vi "OBDservice02.vi"(8 "错误输入（无错误）":errorcluster, 11 "diag ref out输入":T2 {"Diagostic Globals"."Fill Byte" format="%x"; "TesterPresent Message" format="%.0x"; "Selected I/O Mode" items=["CAN", "CAN FD", "CAN FD+BRS", "ECU Determined"]; "DoIP Protocol Version" items=["2010"=1, "2012"=2]; "RX_DL" items=["8"=8, "12"=12, "16"=16, "20"=20, "24"=24, "32"=32, "48"=48, "64"=64]; "TX_DL" items=["8"=8, "12"=12, "16"=16, "20"=20, "24"=24, "32"=32, "48"=48, "64"=64]; "I/O Mode" items=["CAN", "CAN FD", "CAN FD+BRS", "Not yet determined"]}) -> (0 "错误输出":errorcluster, 1 "success?":bool, 2 "冻结帧":T1(array[cluster]), 3 "diag ref out输出":T2 {"Diagostic Globals"."Fill Byte" format="%x"; "TesterPresent Message" format="%.0x"; "Selected I/O Mode" items=["CAN", "CAN FD", "CAN FD+BRS", "ECU Determined"]; "DoIP Protocol Version" items=["2010"=1, "2012"=2]; "RX_DL" items=["8"=8, "12"=12, "16"=16, "20"=20, "24"=24, "32"=32, "48"=48, "64"=64]; "TX_DL" items=["8"=8, "12"=12, "16"=16, "20"=20, "24"=24, "32"=32, "48"=48, "64"=64]; "I/O Mode" items=["CAN", "CAN FD", "CAN FD+BRS", "Not yet determined"]}, 5 "PIDs out":u8[](array[numeric]))   [LabVIEW 2018]
uses:
  <vilib>/Automotive Diagnostic Command Set/Diagnostic Transport.llb/Diag Reference.ctl
  <vilib>/Automotive Diagnostic Command Set/Diagnostic Transport.llb/Transport Protocol Selector.ctl
  <vilib>/Automotive Diagnostic Command Set/Diagnostic Transport.llb/DoIP Protocol Version.ctl
  <vilib>/Automotive Diagnostic Command Set/Diagnostic Transport.llb/Diag Globals.ctl
  <vilib>/Automotive Diagnostic Command Set/Diagnostic Protocols.llb/Diagnostic Trouble Code.ctl
  <vilib>/addons/Automotive Diagnostic Command Set/NI_Automotive Diagnostic Command Set.lvlib
panel:
  out "数组":bool[][](array[boolean])
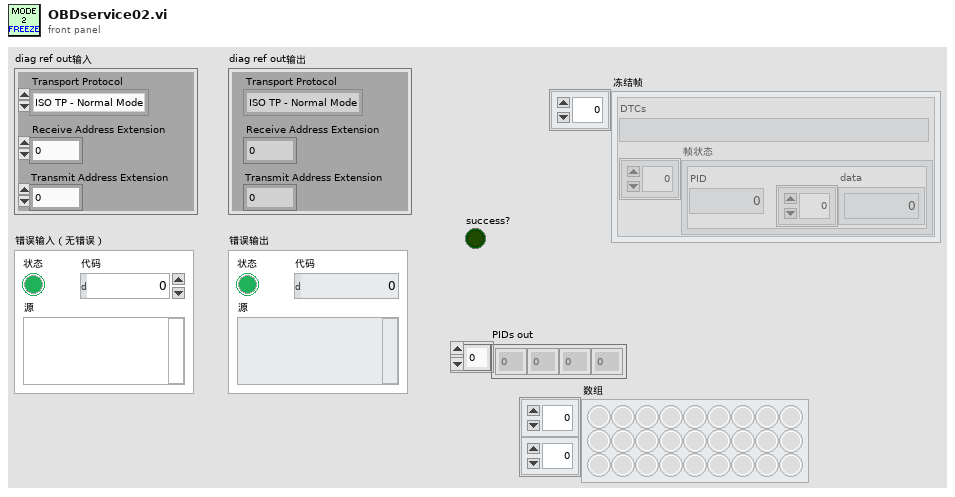
[diagram p1: front panel]
types:
  T1 = cluster{"DTCs":string, "帧状态":cluster{"PID":u8, "data":u8[]}[]}[]
  T2 = typedef "NI_Automotive Diagnostic Command Set.lvlib/Diag Reference.ctl" = cluster{"Diag CAN Handle":u32, "Transport Protocol":T3, "Receive Address Extension":u8, "Transmit Address Extension":u8, "Receive CAN Id":u32, "Transmit CAN Id":u32, "Log Frames ?":bool, "My TP Address":u8, "Other TP Address":u8, "T1":u16, "T2":u16, "T3":u16, "T4":u16, "Tx SN":u8, "Block Size":u8, "Rx SN":u8, "VW TP Initialized?":bool, "Tx block no":u8, "baud rate":u64, "Interface":string, "Channel Diag CAN Handle":u32, "UDP Connection ID":refnum<k16>, "TCP Connection ID":refnum<k5>, "Target IP Addr":u32, "Source Address":u16, "Target Address":u16, "Send Header NACK?":bool, "DLL Handle":u32, "NAD":u8, "Time Stamp read first":dbl, "Time Stamp read last":dbl, "Time Stamp write first":dbl, "Time Stamp write last":dbl, "Time Stamp write":dbl, "Time Stamp read":dbl, " I/O Mode":u32, "FD Baudrate":u64, "TX_DL":u16, "RX_DL":u16, "DoIP Protocol Version":T4, " Selected I/O Mode":u32, "TesterPresent Counter":u32, "TesterPresent Limit":u32, "TesterPresent Tick[ms]":i32, "TesterPresent RequireResponse?":bool, "TesterPresent Stored Ref?":bool, "TesterPresent Message":u8[], "TesterPresent Task Handle":i32, "TesterPresent Semaphore":T5, "Response Plausibility Check":u32, "Default Version?":bool, "Diagostic Globals":T6, "Session-based Properties?":bool}
  T3 = typedef "NI_Automotive Diagnostic Command Set.lvlib/Transport Protocol Selector.ctl" = enum16{"ISO TP - Normal Mode", "ISO TP - Mixed Mode", "VW TP 2.0", "Diagnostics on IP", "ISO TP LIN"}
  T4 = typedef "NI_Automotive Diagnostic Command Set.lvlib/DoIP Protocol Version.ctl" = u8
  T5 = typedef "Semaphore RefNum" = refnum<k1>
  T6 = typedef "NI_Automotive Diagnostic Command Set.lvlib/Diag Globals.ctl" = cluster{"Timeout FC (Bs)":u32, "Timeout CF (Cr)":u32, "Timeout Diag Command":u32, "Receive Block Size (BS)":u8, "Wait Time CF (STmin)":u8, "Max Waits (N_WFTmax)":u8, "Waits to Send (N_WAIT)":i32, "Time between Waits (TW)":u32, "Fill CAN Frames?":bool, "Fill Byte":u32, "Invalid Response as Error?":bool, "Max RspPending Count":u32, "VWTP Command Timeout":u32, "Transport Protocol":T3, "Diag CAN Handle":u32, "DLL Handle":u32, "Timeout RspPending":u32}
  T7 = cluster{"DTCs":string, "数组":cluster{"PID":u8, "data":u8[]}[]}
  T8 = typedef "Diagnostic Trouble Code.ctl" = cluster{"DTC":u32, "Status":u32, "Add Data":u32}
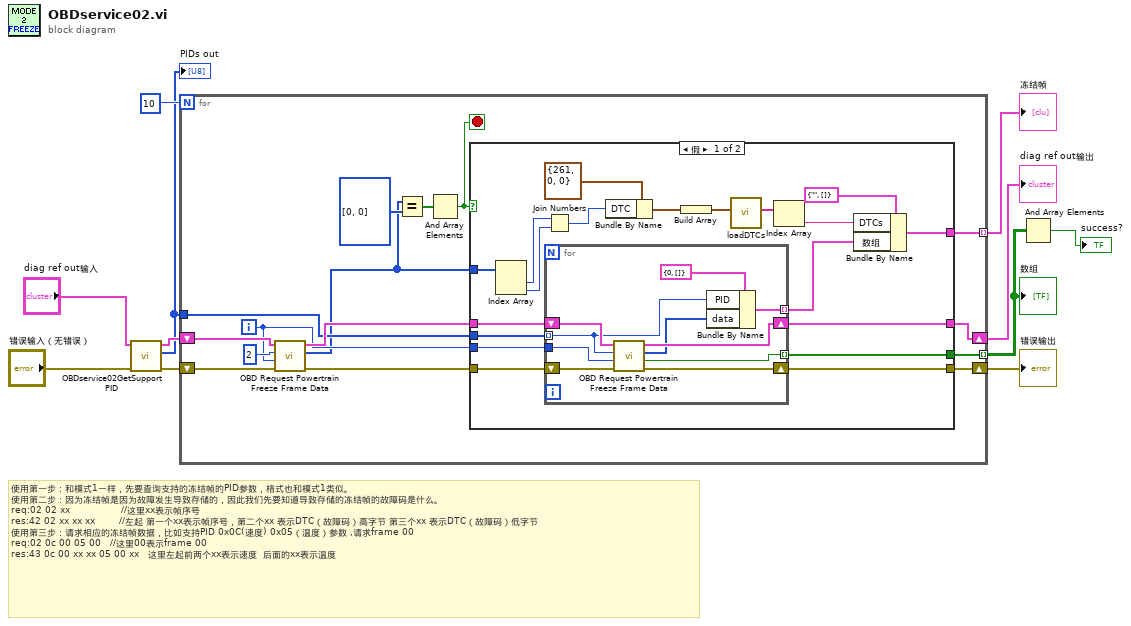
[diagram p0: block diagram]
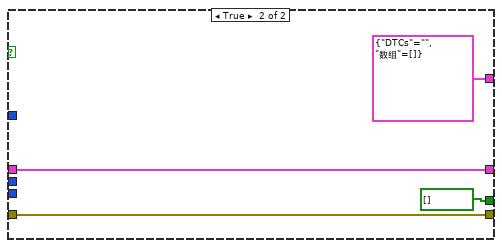
[diagram p2: hidden frame]
diagram:
  # "使用第一步：和模式1一样，先要查询支持的冻结帧的PID参数，格式也和模式1类似。\n使用第二步：因为冻结帧是因为故障发生导致存储的，因此我们先要知道导致存储的冻结帧的故障码是什么。\nreq:02 02 xx                 //这里xx表示帧序号\nres:42 02 xx xx xx        //左起 第一个xx表示帧序号，第二个xx 表示DTC（故障码）高字节 第三个xx 表示DTC（故障码）低字节\n使用第三步：请求相应的冻结帧数据，比如支持PID 0x0C(速度) 0x05（温度）参数 ,请求frame 00\nreq:02 0c 00 05 00   //这里00表示frame 00 \nres:43 0c 00 xx xx 05 00 xx   这里左起前两个xx表示速度  后面的xx表示温度"
  n1 = call "OBDservice02GetSupportPID.vi"("error in (no error) 2"="错误输入（无错误）", "diag ref in"="diag ref out输入") -> ("error out 2"=w8:errorcluster, "PIDs out"=w6:u8[], "diag ref out 2"=w9:T2)  [unwired: 6 in, 1 out]
  "PIDs out" <- w6
  n2 = for {
    N: 10 -> [_]
    tunnel: w6 -> [w20]
    shift-right: [w19] -> w5
    shift-left: w9 -> [w26]
    tunnel: [w18] -> w4 mode=indexing
    shift-right: [w17] -> w2
    shift-left: w8 -> [w24]
    tunnel: [w14] -> w1 mode=indexing
    i -> [w21]
    stop <- w13 stop-if-true
    n3 = call <vilib>:"OBD Request Powertrain Freeze Frame Data.vi"("error in (no error)"=w24, "# frame"=w21, "PID"=u8 2, "diag ref in"=w26) -> ("error out"=w22:errorcluster, "data out"=w12:u8[], "diag ref out"=w23:T2)  [unwired: 4 in, 1 out]
    n4 = Equal?(x=w12, y=u8[] [0, 0]) -> (x = y?=w15:bool[])
    n5 = And Array Elements(Boolean array=w15) -> (logical AND=w13:bool)
    n6 = case shown="假" w13 {
      tunnel: w23 -> [w45 w59]
      tunnel: w22 -> [w44 w56]
      tunnel: w21 -> [w43 _]
      tunnel: w20 -> [w42 _]
      tunnel: [w41 w59] -> w19
      tunnel: [w40 bool[] []] -> w18
      tunnel: [w39 w56] -> w17
      tunnel: w12 -> [w34 _]
      tunnel: [w28 T7 {"DTCs"="", "数组"=[]} ("簇 2")] -> w14
      frame False {
        n7 = Index Array(array=w34) -> (element #1=w36:u8, element #2=w35:u8)  [unwired: 2 in]
        n8 = Join Numbers(hi=w36, lo=w35) -> ((hi.lo)=w37:u16)
        n9 = for {
          tunnel: w43 -> [w53]
          tunnel: w42 -> [w48] mode=indexing
          shift-right: [w52] -> w41
          shift-left: w45 -> [w55]
          tunnel: [w51] -> w40 mode=indexing
          shift-right: [w50] -> w39
          shift-left: w44 -> [w54]
          tunnel: [w46] -> w29 mode=indexing
          n10 = call <vilib>:"OBD Request Powertrain Freeze Frame Data.vi"("error in (no error)"=w54, "# frame"=w53, "PID"=w48, "diag ref in"=w55) -> ("error out"=w50:errorcluster, "success?"=w51:bool, "data out"=w47:u8[], "diag ref out"=w52:T2)  [unwired: 4 in]
          n11 = Bundle By Name(cluster=cluster{"PID":u8, "data":u8[]} {"PID"=0, "data"=[]} ("冻结帧内容"), "PID"=w48, "data"=w47) -> (w46:cluster{"PID":u8, "data":u8[]})
        }
        n12 = Bundle By Name(cluster=T8 {"DTC"=261, "Status"=0, "Add Data"=0} ("Diagnostic Trouble Code"), "DTC"=w37) -> (w33:T8)
        n13 = Build Array(w33) -> (w32:T8[])
        n14 = call "loadDTCs.vi"("DTCs"=w32) -> ("dtcs"=w31:string[])  [unwired: 10 in]
        n15 = Index Array(array=w31) -> (element=w30:string)  [unwired: 1 in]
        n16 = Bundle By Name(cluster=T7 {"DTCs"="", "数组"=[]} ("簇 2"), "DTCs"=w30, "数组"=w29) -> (w28:T7)
      }
      frame True {
      }
    }
  }
  "错误输出" <- w2
  "diag ref out输出" <- w5
  "冻结帧" <- w1
  "数组" <- w4
  n17 = And Array Elements(Boolean array=w4) -> (logical AND=→"success?":bool)
